vi "evo irimager set radiation parameters.vi"(9 "tAmbient":sgl, 10 "transmissivity":sgl, 11 "emissivity":sgl) -> (3 "function return":i32)   [LabVIEW 2025, in "libirimager_direct_binding.lvlib"]
doc: "__IRDIRECTSDK_API__ int evo_irimager_set_radiation_parameters(float emissivity, float transmissivity, float tAmbient=-999.f);"
uses:
  libirimager_direct_binding.lvlib
  libirimager.dll
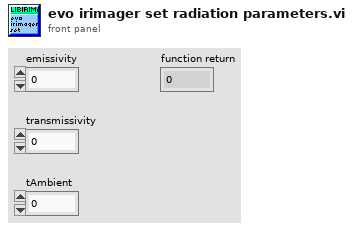
[diagram p1: front panel]
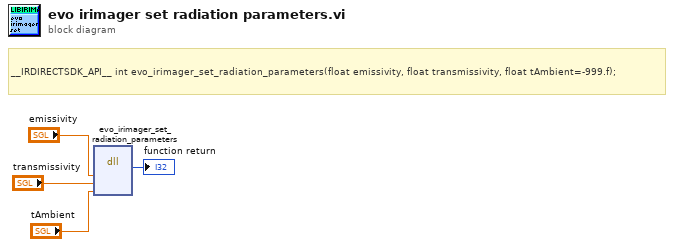
[diagram p0: block diagram]
diagram:
  # "__IRDIRECTSDK_API__ int evo_irimager_set_radiation_parameters(float emissivity, float transmissivity, float tAmbient=-999.f);"
  n1 = dll-call lib="C:/Users/mayhe/OneDrive/Documents/GitHub/In-situ-monitoring-of-powder-bed-fusion-additive-manufacturing/system_development/Orichalcum/v0.2/Software_design/thermal-camera/VI/labview/libirimager.dll" fn="evo_irimager_set_radiation_parameters"("emissivity"="emissivity", "transmissivity"="transmissivity", "tAmbient"="tAmbient") -> ("Rückgabetyp"=→"function return":i32)  [unwired: 6 in, 2 out]
